vi "Movimiento Motor.vi"(11 "Configuracion Movimiento":string) -> ()   [LabVIEW 2013, in "Proyecto 2 Touch.lvrbt"]
uses:
  Proyecto 2 Touch.lvrbt
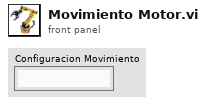
[diagram p1: front panel]
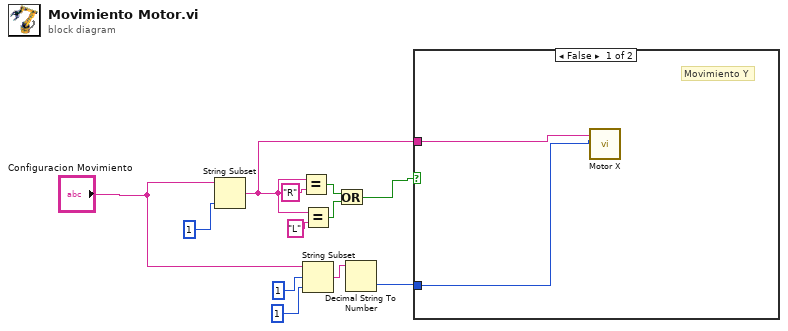
[diagram p0: block diagram]
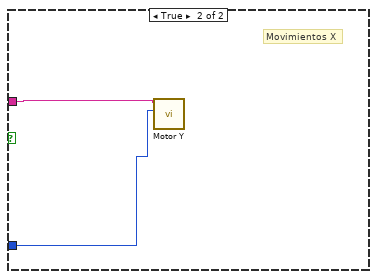
[diagram p2: hidden frame]
diagram:
  n1 = String Subset(string="Configuracion Movimiento", length (rest)=1 ("length (rest)")) -> (substring=w1:string)  [unwired: 1 in]
  n2 = Equal?(x=w1, y="R") -> (x = y?=w10:bool)
  n3 = Equal?(x=w1, y="L") -> (x = y?=w9:bool)
  n4 = String Subset(string="Configuracion Movimiento", offset (0)=1, length (rest)=1 ("length (rest)")) -> (substring=w5:string)
  n5 = Or(x=w10, y=w9) -> (x .or. y?=w7:bool)
  n6 = Decimal String To Number(string=w5) -> (number=w4:i32)  [unwired: 2 in, 1 out]
  n7 = case shown="False" w7 {
    tunnel: w4 -> [w13 w15]
    tunnel: w1 -> [w14 w16]
    frame False {
      # "Movimiento Y"
      n8 = call "Motor X.vi"("Magnitud Movimiento"=w13, "Direccion Movimiento"=w14) -> ()  [unwired: 10 in]
    }
    frame True {
      # "Movimientos X"
      n9 = call "Motor Y.vi"("Magnitud Movimiento"=w15, "Direccion Movimiento"=w16) -> ()  [unwired: 10 in]
    }
  }
